vi "Example1.vi"() -> ()   [LabVIEW 2011]
uses:
  Interprocess Messenger/QueueMessenger/QueueMessenger.lvclass
  Interprocess Messenger/TextVarientMessage/MSG.lvclass
  Interprocess Messenger/TextVarientMessage/Extract Text (static).vi
  Interprocess Messenger/TextVarientMessage/Write (no data).vi
  Interprocess Messenger/Send/Send.lvclass
  Interprocess Messenger/Send/Send Message.vi
  Interprocess Messenger/Send/Send (no data).vi
  Interprocess Messenger/SendOnly/Observer.lvclass
  Interprocess Messenger/TextVarientMessage/Reply (varient).vi
panel:
  out "Time":string
  # "Any Key Down to stop"
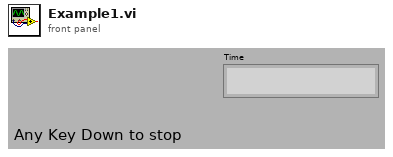
[diagram p1: front panel]
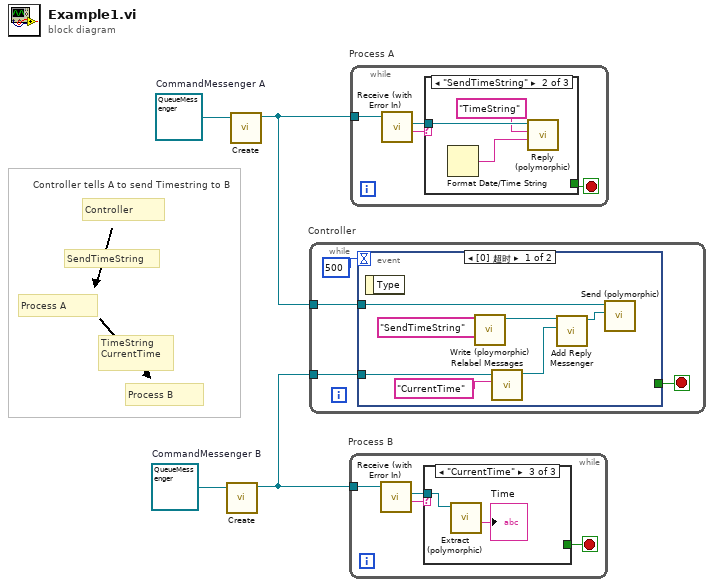
[diagram p0: block diagram]
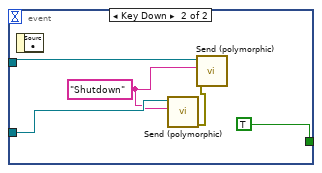
[diagram p2: hidden frame]
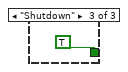
[diagram p4: hidden frame]
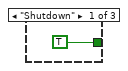
[diagram p5: hidden frame]
diagram:
  w3 = refnum<class "QueueMessenger.lvclass"> refnum  # CommandMessenger A
  w4 = refnum<class "QueueMessenger.lvclass"> refnum  # CommandMessenger B
  # "TimeString \nCurrentTime"
  # "Controller tells A to send Timestring to B"
  # "SendTimeString"
  # "Process B"
  # "Process A"
  # "Controller"
  n1 = call-dynamic "Create.vi"("QueueMessenger in"=w4) -> ("QueueMessenger out"=w1:refnum<class "QueueMessenger.lvclass">)  [unwired: 1 in, 9 out]
  n2 = call-dynamic "Create.vi"("QueueMessenger in"=w3) -> ("QueueMessenger out"=w2:refnum<class "QueueMessenger.lvclass">)  [unwired: 1 in, 9 out]
  n3 = while "Controller" {
    tunnel: w2 -> [w8]
    tunnel: w1 -> [w7]
    stop <- w6 stop-if-true
    n4 = event shown="[0] 超时" {
      selector: _ -> [_ _]
      dyn-events: _ -> [_ _]
      timeout: 500 -> [_ _]
      tunnel: w8 -> [w12 w19]
      tunnel: w7 -> [w11 w17]
      tunnel: [_ TRUE] -> w6
      event Timeout {
        n5 = event-data() -> ()  [unwired: 2 out]
        n6 = call-poly "Write (ploymorphic).vi"("Label"="SendTimeString") -> ("Message"=w14:refnum<class "MSG.lvclass">)  [unwired: 1 in, 9 out]
        n7 = call "Relabel Messages.vi"("Relabel messages with"="CurrentTime" ("Reply Label"), "Send IN"=w11) -> ("Observer"=w10:refnum<class "Observer.lvclass">)  [unwired: 9 out]
        n8 = call "Add Reply Messenger.vi"("Reply to..."=w10, "Message"=w14) -> ("Message"=w15:refnum<class "MSG.lvclass">)  [unwired: 2 in, 7 out]
        n9 = call-poly "Send (polymorphic).vi"("Message"=w15, "MSR Parent in"=w12) -> ()  [unwired: 1 in, 9 out]
      }
      event Key Down {
        w16 = "Shutdown"
        n10 = event-data() -> ()  [unwired: 2 out]
        n11 = call-poly "Send (polymorphic).vi"("Label"=w16, "MSR Parent in"=w17) -> ("error out"=w18:errorcluster)  [unwired: 1 in, 8 out]
        n12 = call-poly "Send (polymorphic).vi"("error in (no error)"=w18, "Label"=w16, "MSR Parent in"=w19) -> ()  [unwired: 9 out]
      }
    }
  }
  n13 = while "Process B" {
    tunnel: w1 -> [w24]
    stop <- w21 stop-if-true
    n14 = call-dynamic "Receive (with Error In).vi"("MGR in"=w24) -> ("Label"=w23:string, "Message"=w22:refnum<class "MSG.lvclass">)  [unwired: 2 in, 7 out]
    n15 = case shown="\"CurrentTime\"" w23 {
      tunnel: w22 -> [_ _ w27]
      tunnel: [TRUE _ _] -> w21
      frame "Shutdown" {
      }
      frame Default {
      }
      frame "CurrentTime" {
        n16 = call-poly "Extract (polymorphic).vi"("TextMessage in"=w27) -> ("Text"=→"Time":string)  [unwired: 1 in, 9 out]
      }
    }
  }
  n17 = while "Process A" {
    tunnel: w2 -> [w31]
    stop <- w28 stop-if-true
    n18 = call-dynamic "Receive (with Error In).vi"("MGR in"=w31) -> ("Label"=w30:string, "Message"=w29:refnum<class "MSG.lvclass">)  [unwired: 2 in, 7 out]
    n19 = case shown="\"SendTimeString\"" w30 {
      tunnel: w29 -> [_ w34 _]
      tunnel: [_ _ TRUE] -> w28
      frame "False", Default {
      }
      frame "SendTimeString" {
        n20 = Format Date/Time String() -> (date/time string=w32:string)  [unwired: 3 out]
        n21 = call-poly "Reply (polymorphic).vi"("Varient"=w32, "Reply"="TimeString", "Message to Reply to"=w34) -> ()  [unwired: 1 in, 8 out]
      }
      frame "Shutdown" {
      }
    }
  }
